vi "gyro -- sourcer async - V3 -- arydh.vi"(11 "sourcer event pair":T8) -> ()   [LabVIEW 2018]
uses:
  publisher action.ctl
  MFLI frontend action.ctl
  mfli reader event.ctl
  server talkto message type.ctl
  data source action.ctl
  PLL data source.ctl
  nanocal/Nanocalorimetry/data/MCL.lvlibp/SynkTek FPGA/FPGA_SharedResources/FPGASharedResources_Lockin_Typedef.ctl
  server talk-to-back pair.ctl
  server talkback message type.ctl
  nanocal/Nanocalorimetry/data/MCL.lvlibp/SynkTek FPGA/FPGA_SharedResources/FPGASharedResources_FreqCtrl_FreqGenTypedef.ctl
  nanocal/Nanocalorimetry/data/MCL.lvlibp/SynkTek Host/LIControl/LIControl_LockinTimeConstant_typedef.ctl
  nanocal/Nanocalorimetry/data/MCL.lvlibp/SynkTek FPGA/FPGA_SharedResources/FPGASharedResources_HarmonicTypdef.ctl
  nanocal/Nanocalorimetry/data/MCL.lvlibp/SynkTek FPGA/FPGA_SharedResources/FPGASharedResources_LockinTypeTypedef.ctl
  nanocal/Nanocalorimetry/data/MCL.lvlibp/SynkTek FPGA/FPGA_SharedResources/FPGASharedResources_PhaseShiftCtrl_Typedef.ctl
  nanocal/Nanocalorimetry/data/MCL.lvlibp/SynkTek FPGA/FPGA_SharedResources/FPGASharedResources_DutyCycleCtrl_Typedef.ctl
  nanocal/Nanocalorimetry/data/MCL.lvlibp/SynkTek Host/LIControl/LIControl_LockinCtrl_typedef.ctl
panel:
  in  "LockinCtrl":T1={"Frequency generator"=enum."Frequency 1", "Time constant (s)"=1.0, "Exponential low-pass filter"={"Enabled"=TRUE, "Stage 1 time const. (s)"=0.3, "Stage 2 time const. (s)"=0.1}, "Harmonic"=1, "Type"=enum."Sine", "Phase shift"=enum."Phase 1", "Duty cycle"=enum."DutyCycle 1"} {"Exponential low-pass filter"."Stage 2 time const. (s)" items=["100 s"=100.0, "50 s"=50.0, "20 s"=20.0, "10 s"=10.0, "5 s"=5.0, "3 s"=3.0, "2 s"=2.0, "1 s"=1.0, "0.5 s"=0.5, "0.3 s"=0.3, "0.2 s"=0.2, "0.1 s"=0.1, "50 ms"=0.05, "20 ms"=0.02, "10 ms"=0.01, "5 ms"=0.005, "2 ms"=0.002, "1 ms"=0.001]; "Exponential low-pass filter"."Stage 1 time const. (s)" items=["100 s"=100.0, "50 s"=50.0, "20 s"=20.0, "10 s"=10.0, "5 s"=5.0, "3 s"=3.0, "2 s"=2.0, "1 s"=1.0, "0.5 s"=0.5, "0.3 s"=0.3, "0.2 s"=0.2, "0.1 s"=0.1, "50 ms"=0.05, "20 ms"=0.02, "10 ms"=0.01, "5 ms"=0.005, "2 ms"=0.002, "1 ms"=0.001]; "Time constant (s)" items=["100 s"=100.0, "50 s"=50.0, "20 s"=20.0, "10 s"=10.0, "5 s"=5.0, "3 s"=3.0, "2 s"=2.0, "1 s"=1.0, "0.5 s"=0.5, "0.3 s"=0.3, "0.2 s"=0.2, "0.1 s"=0.1, "50 ms"=0.05, "20 ms"=0.02, "10 ms"=0.01, "5 ms"=0.005, "2 ms"=0.002, "1 ms"=0.001]}
  in  "all":enum32{"all", "all 2"}(tab)
  out "read Voltage (V)":cdb=2.0706635468928775e-07+4.4716444398634134e-07i format="%#10_10f"
  in  "read status":bool
  out "read Voltage X (V)":dbl=2.0706635468928775e-07 format="%#11_11f"
  out "read Voltage Y (V)":dbl=4.4716444398634134e-07 format="%#11_11f"
  in  "delay-read (msec)":i64=20
  out "zi freq (Hz)":dbl=99999.99999990905 format="%-#.3f"
  in  "amplitude (V)":dbl=0.01
  in  "set amp! :m":bool
  in  "start  !":bool
  in  "stop  !":bool
  out "device selector":enum32{"MFLI", "ARydh", "meta"}(tab)
  out "Stopped?":bool=TRUE
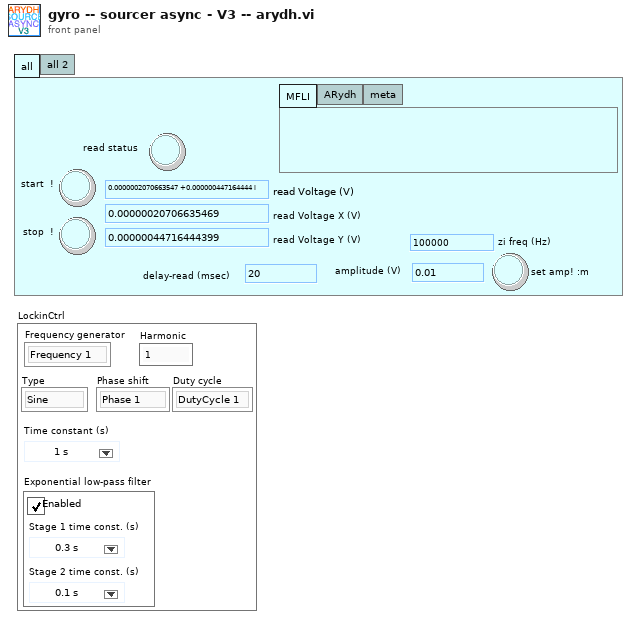
[diagram p1: front panel]
types:
  T1 = typedef "MCL.lvlibp/LIControl.lvlib/LIControl_LockinCtrl_typedef.ctl" = cluster{"Frequency generator":T2, "Time constant (s)":T3, "Exponential low-pass filter":cluster{"Enabled":bool, "Stage 1 time const. (s)":T3, "Stage 2 time const. (s)":T3}, "Harmonic":T4, "Type":T5, "Phase shift":T6, "Duty cycle":T7}
  T2 = typedef "MCL.lvlibp/FPGA_SharedResources.lvlib/FPGASharedResources_FreqCtrl_FreqGenTypedef.ctl" = enum8{"Frequency 1", "Frequency 2", "Frequency 3", "Frequency 4", "Frequency 5", "Frequency 6: PLL 1", "Frequency 7: PLL 2", "Frequency 8"}
  T3 = typedef "MCL.lvlibp/LIControl.lvlib/LIControl_LockinTimeConstant_typedef.ctl" = dbl
  T4 = typedef "MCL.lvlibp/FPGA_SharedResources.lvlib/FPGASharedResources_HarmonicTypdef.ctl" = u16
  T5 = typedef "MCL.lvlibp/FPGA_SharedResources.lvlib/FPGASharedResources_LockinTypeTypedef.ctl" = enum8{"Sine", "Square", "Boxcar"}
  T6 = typedef "MCL.lvlibp/FPGA_SharedResources.lvlib/FPGASharedResources_PhaseShiftCtrl_Typedef.ctl" = enum8{"Phase 1", "Phase 2", "Phase 3", "Phase 4", "Phase 5", "Phase 6", "Phase 7", "Disabled"}
  T7 = typedef "MCL.lvlibp/FPGA_SharedResources.lvlib/FPGASharedResources_DutyCycleCtrl_Typedef.ctl" = enum8{"DutyCycle 1", "DutyCycle 2", "DutyCycle 3", "DutyCycle 4", "DutyCycle 5", "DutyCycle 6", "DutyCycle 7", "Inactive"}
  T8 = typedef "server talk-to-back pair.ctl" = cluster{"talkback event":refnum<user-event>, "talkto event":refnum<user-event>}
  T9 = typedef "PLL data source.ctl" = enum16{"meta", "MFLI", "SRS865A", "arydh"}
  T10 = typedef "server talkto message type.ctl" = cluster{"message":enum16{"stop", "start", "update pars", "update request", "new", "launch", "exit", "get", "reset", "pause", "unpause"}}
  T11 = typedef "mfli reader event.ctl" = enum16{"start", "stop", "exit", "set amplitude", "set datarate"}
  T12 = typedef "MFLI frontend action.ctl" = enum16{"read", "writeread", "open", "close", "write"}
  T13 = typedef "publisher action.ctl" = enum16{"set", "get", "init", "check"}
  T14 = typedef "MCL.lvlibp/FPGA_SharedResources.lvlib/FPGASharedResources_Lockin_Typedef.ctl" = enum8{"Lock-in set L1", "Lock-in set L2"}
  T15 = typedef "data source action.ctl" = enum16{"set", "get", "init", "set-and-get", "init source"}
  T16 = typedef "Zurich Instruments LabOne.lvlib/ziTypeHandle.ctl" = cluster{"handleValid":bool, "Conn":u64, "Path Prefix":string, "Handle":u64, "Connected":bool, "Clockbase(s)":dbl}
  T17 = typedef "MCL.lvlibp/MCL_DataRef.ctl" = refnum<vi>
  T18 = enum16{"stop", "start", "update pars", "update request", "new", "launch", "exit", "get", "reset", "pause", "unpause"}
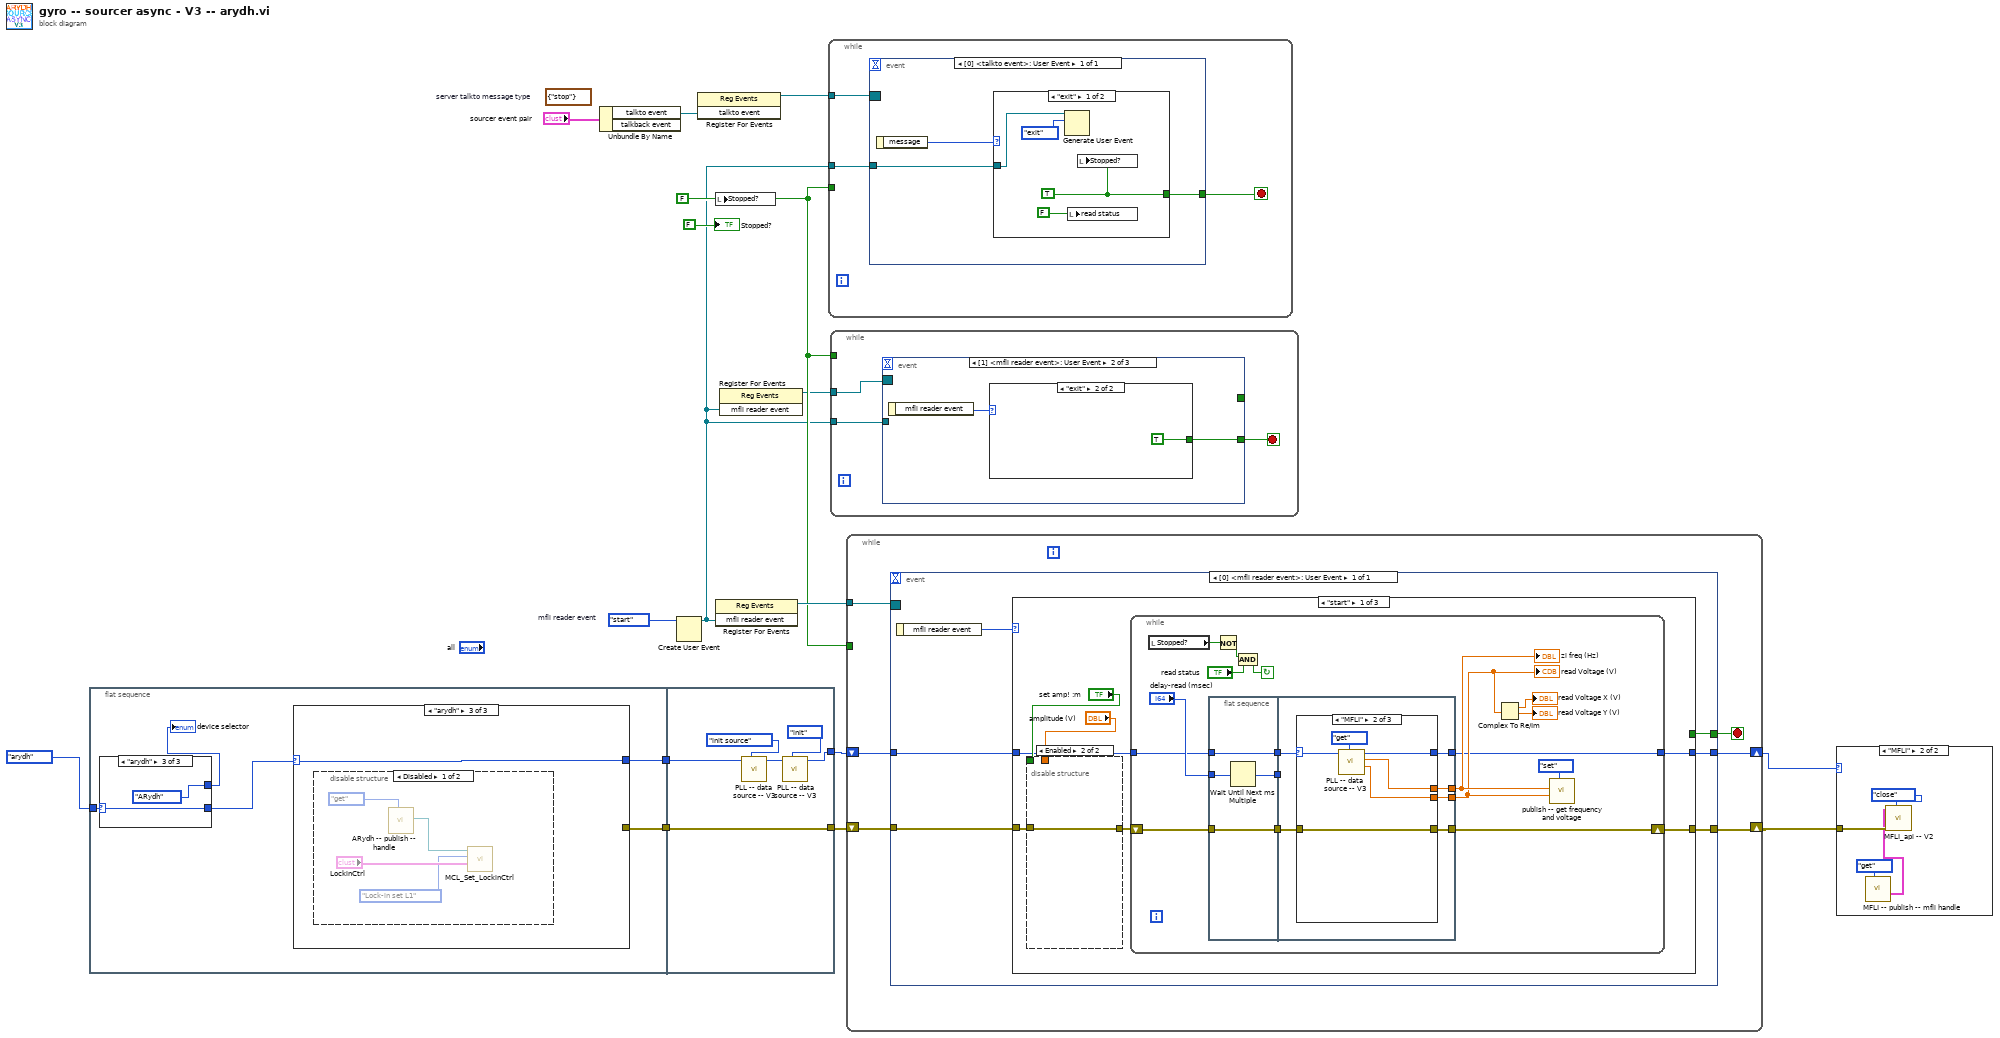
[diagram p0: block diagram]
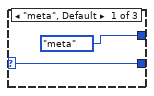
[diagram p3: hidden frame]
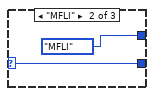
[diagram p4: hidden frame]
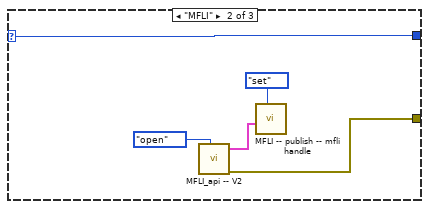
[diagram p6: hidden frame]
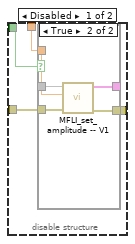
[diagram p9: hidden frame]
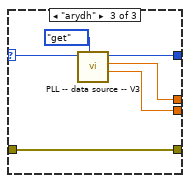
[diagram p12: hidden frame]
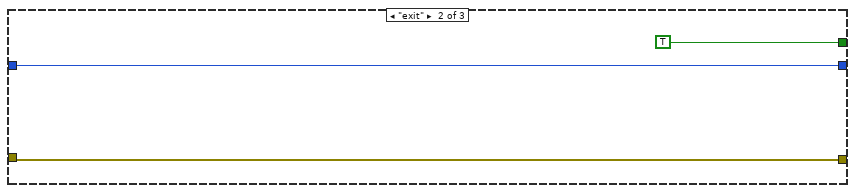
[diagram p13: hidden frame]
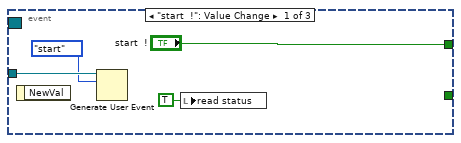
[diagram p15: hidden frame]
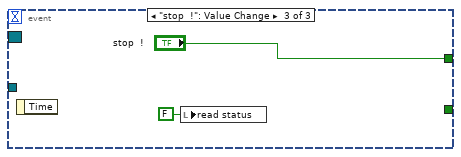
[diagram p17: hidden frame]
diagram:
  (unwired) T10 {"message"=enum."stop"}  # server talkto message type
  w7 = FALSE ("Stop")
  w15 = mfli_reader_event."start"  # mfli reader event
  n1 = flat-sequence {
    tunnel: [w21] -> w8
    tunnel: PLL_data_source."arydh" ("PLL data source") -> [w20]
    tunnel: [w18] -> w3
    tunnel: [w45] -> w13
    tunnel: w8 -> [w45]
    tunnel: w3 -> [w42]
    tunnel: [w40] -> w2
    frame #0 {
      n2 = case shown="\"arydh\"" w20 {
        selector: w20 -> [w23 w25 w27]
        tunnel: [enum32{"MFLI", "ARydh", "meta"}."meta" ("device selector") enum32{"MFLI", "ARydh", "meta"}."MFLI" ("device selector") enum32{"MFLI", "ARydh", "meta"}."ARydh" ("device selector")] -> w17
        tunnel: [w23 w25 w27] -> w19
        frame "meta", Default {
        }
        frame "MFLI" {
        }
        frame "arydh" {
        }
      }
      "device selector" <- w17
      n3 = case shown="\"arydh\"" w19 {
        selector: w19 -> [w28 w29 w34]
        tunnel: [_ w30 _] -> w21
        tunnel: [w28 w29 w34] -> w18
        frame "meta", Default {
        }
        frame "MFLI" {
          n4 = call "MFLI_api -- V2.vi"("MFLI frontend action"=MFLI_frontend_action."open") -> ("Error Out"=w30:errorcluster, "Handle Out"=w31:T16)  [unwired: 7 in, 2 out]
          n5 = call "MFLI -- publish -- mfli handle.vi"("publisher action"=publisher_action."set", "Handle IN"=w31) -> ()  [unwired: 9 in, 1 out]
        }
        frame "arydh" {
          n6 = disable-structure shown="Disabled" {
            frame Disabled {
              n7 = call "ARydh -- publish -- handle.vi"("publisher action"=publisher_action."get") -> ("MCL object OUT"=w36:T17)  [unwired: 10 in]
              n8 = call "MCL_Set_LockinCtrl.vi"("LockinCtrl"="LockinCtrl", "Lockin"=FPGASharedResources_Lockin_Typedef."Lock-in set L1", "MCL object"=w36) -> ()  [unwired: 3 in, 2 out]
            }
            frame Enabled {
            }
          }
        }
      }
    }
    frame #1 {
      n9 = call "PLL -- data source -- V3.vi"("data source action"=data_source_action."init source", "PLL data source"=w42) -> ("PLL data source OUT"=w44:T9)  [unwired: 7 in, 2 out]
      n10 = call "PLL -- data source -- V3.vi"("data source action"=data_source_action."init", "PLL data source"=w44) -> ("PLL data source OUT"=w40:T9, 4:w39)  [unwired: 6 in, 2 out]
    }
  }
  n11 = Unbundle By Name("sourcer event pair") -> ("talkto event"=w10:refnum<user-event>)  [unwired: 1 out]
  n12 = Create User Event(user event datatype=w15) -> (user event=w5:refnum<user-event>)  [unwired: 1 in, 1 out]
  n13 = register-events(w10) -> (reference out=w12:refnum<event-registration>)  [unwired: 2 in, 1 out]
  n14 = local write "Stopped?"(w7) -> ()
  n15 = register-events(w5) -> (reference out=w16:refnum<event-registration>)  [unwired: 2 in, 1 out]
  n16 = register-events(w5) -> (reference out=w6:refnum<event-registration>)  [unwired: 2 in, 1 out]
  n17 = while {
    tunnel: w12 -> [w48]
    tunnel: w7 -> [_]
    tunnel: w5 -> [w46]
    stop <- w47 stop-if-true
    n18 = event shown="[0] <talkto event>: User Event" {
      selector: w48 -> [_]
      dyn-events: _ -> [_]
      timeout: _ -> [_]
      tunnel: [w50] -> w47
      tunnel: w46 -> [w49]
      event User Event {
        n19 = event-data() -> ("message"=w51:T18)  [unwired: 1 in]
        n20 = case shown="\"exit\"" w51 {
          tunnel: [w54 _] -> w50
          tunnel: w49 -> [w53 _]
          frame "exit" {
            w54 = TRUE ("Stoped?")
            n21 = Generate User Event(user event=w53, event data cluster=mfli_reader_event."exit" ("event data")) -> ()  [unwired: 2 in, 2 out]
            n22 = local write "read status"(FALSE ("read status")) -> ()
            n23 = local write "Stopped?"(w54) -> ()
          }
          frame "get", Default {
          }
        }
      }
    }
  }
  n24 = while {
    tunnel: w5 -> [w58]
    tunnel: w7 -> [_]
    tunnel: w6 -> [w57]
    stop <- w56 stop-if-true
    n25 = event shown="[1] <mfli reader event>: User Event" {
      selector: w57 -> [_ _ _]
      dyn-events: _ -> [_ _ _]
      timeout: _ -> [_ _ _]
      tunnel: ["start  !" _ "stop  !"] -> _
      tunnel: w58 -> [w60 _ _]
      tunnel: [_ w63 _] -> w56
      event "start  !": Value Change {
        n26 = event-data() -> ()  [unwired: 1 in, 1 out]
        n27 = Generate User Event(user event=w60, event data cluster=mfli_reader_event."start" ("event data")) -> ()  [unwired: 2 in, 2 out]
        n28 = local write "read status"(TRUE ("read status")) -> ()
      }
      event User Event {
        n29 = event-data() -> ("mfli reader event"=w64:T11)  [unwired: 1 in]
        n30 = case shown="\"exit\"" w64 {
          tunnel: [_ TRUE] -> w63
          frame "start", Default {
          }
          frame "exit" {
          }
        }
      }
      event "stop  !": Value Change {
        n31 = event-data() -> ()  [unwired: 1 in, 1 out]
        n32 = local write "read status"(FALSE ("read status")) -> ()
      }
    }
  }
  n33 = while {
    tunnel: w16 -> [w73]
    shift-right: [w72] -> w14
    shift-left: w13 -> [w71]
    tunnel: w7 -> [_]
    shift-right: [w68] -> w1
    shift-left: w2 -> [w69]
    stop <- w70 stop-if-true
    n34 = event shown="[0] <mfli reader event>: User Event" {
      selector: w73 -> [_]
      dyn-events: _ -> [_]
      timeout: _ -> [_]
      tunnel: w71 -> [w79]
      tunnel: [w78] -> w72
      tunnel: [w76] -> w70
      tunnel: w69 -> [w75]
      tunnel: [w74] -> w68
      event User Event {
        n35 = event-data() -> ("mfli reader event"=w77:T11)  [unwired: 1 in]
        n36 = case shown="\"start\"" w77 {
          tunnel: w79 -> [w85 w142 w144]
          tunnel: [w82 w142 w144] -> w78
          tunnel: [_ TRUE _] -> w76
          tunnel: w75 -> [w81 w140 w143]
          tunnel: [w80 w140 w143] -> w74
          frame "start" {
            n37 = disable-structure shown="Enabled" {
              disable-tunnel: "set amp! :m" -> [w90 _]
              disable-tunnel: w85 -> [w89 w98]
              disable-tunnel: [w88 w98] -> w84
              disable-tunnel: "amplitude (V)" -> [w87 _]
              frame Disabled {
                n38 = case shown="True" w90 {
                  tunnel: _ -> [w92 w97]
                  tunnel: [w92 w96] -> _
                  tunnel: w89 -> [w91 w95]
                  tunnel: [w91 w94] -> w88
                  tunnel: w87 -> [_ w93]
                  frame False {
                  }
                  frame True {
                    n39 = call "MFLI_set_amplitude -- V1.vi"("Error In"=w95, "Amp in (V)"=w93, "Handle In"=w97) -> ("Error Out"=w94:errorcluster, "Handle Out"=w96:T16)  [unwired: 5 in, 2 out]
                  }
                }
              }
              frame Enabled {
              }
            }
            n40 = while {
              shift-right: [w114] -> w82
              shift-left: w84 -> [w115]
              tunnel: w81 -> [w99]
              tunnel: [w101] -> w80
              stop <- w104 continue-if-true
              n41 = local read "Stopped?"() -> (w102:bool)
              n42 = flat-sequence {
                tunnel: [w119] -> w113
                tunnel: "delay-read (msec)" -> [w118]
                tunnel: [w117] -> w112
                tunnel: w115 -> [w117]
                tunnel: [w116] -> w100
                tunnel: w99 -> [w116]
                tunnel: w113 -> [_]
                tunnel: [w123] -> w106
                tunnel: [w122] -> w107
                tunnel: w112 -> [w125]
                tunnel: [w124] -> w114
                tunnel: [w121] -> w101
                tunnel: w100 -> [w120]
                frame #0 {
                  n43 = Wait Until Next ms Multiple(millisecond multiple=w118) -> (millisecond timer value=w119:u32)
                }
                frame #1 {
                  n44 = case shown="\"MFLI\"" w120 {
                    selector: w120 -> [w126 w133 w139]
                    tunnel: w125 -> [w127 w130 w137]
                    tunnel: [w127 w130 w137] -> w124
                    tunnel: [_ w129 w135] -> w123
                    tunnel: [_ w128 w136] -> w122
                    tunnel: [w126 w132 w134] -> w121
                    frame "meta", Default {
                    }
                    frame "MFLI" {
                      n45 = call "PLL -- data source -- V3.vi"("data source action"=data_source_action."get", "PLL data source"=w133) -> ("z out (V)"=w129:cdb, "Freq out (Hz)"=w128:dbl, "PLL data source OUT"=w132:T9)  [unwired: 7 in]
                    }
                    frame "arydh" {
                      n46 = call "PLL -- data source -- V3.vi"("data source action"=data_source_action."get", "PLL data source"=w139) -> ("z out (V)"=w135:cdb, "Freq out (Hz)"=w136:dbl, "PLL data source OUT"=w134:T9)  [unwired: 7 in]
                    }
                  }
                }
              }
              n47 = Not(x=w102) -> (.not. x?=w105:bool)
              n48 = And(x=w105, y="read status") -> (x .and. y?=w104:bool)
              n49 = Complex To Re/Im(x + iy=w106) -> (x=→"read Voltage X (V)":dbl, y=→"read Voltage Y (V)":dbl)
              n50 = call "publish -- get frequency and voltage.vi"("publisher action"=publisher_action."set", "Voltage IN (V)"=w106, "freq IN (Hz)"=w107) -> ()  [unwired: 6 in, 3 out]
              "read Voltage (V)" <- w106
              "zi freq (Hz)" <- w107
            }
          }
          frame "exit" {
          }
          frame "stop", Default {
          }
        }
      }
    }
  }
  n51 = case shown="\"MFLI\"" w1 {
    tunnel: w14 -> [_ w148]
    frame "meta", Default {
    }
    frame "MFLI" {
      n52 = call "MFLI -- publish -- mfli handle.vi"("publisher action"=publisher_action."get") -> ("Handle Out"=w145:T16)  [unwired: 10 in]
      n53 = call "MFLI_api -- V2.vi"("MFLI frontend action"=MFLI_frontend_action."close", "Error In"=w148, "Handle In"=w145) -> ()  [unwired: 5 in, 4 out]
    }
  }
  "Stopped?" <- FALSE ("Stoped?")
